vi "Perform Action.vi"(8 "error in":errorcluster, 10 "Input":variant, 11 "Red-y Read Write CFG in":refnum<class "Red-y Pressure Control CFG Simulated.lvclass">) -> (0 "error out":errorcluster, 2 "Output":variant, 3 "Red-y Read Write CFG out":refnum<class "Red-y Pressure Control CFG Simulated.lvclass">)   [LabVIEW 2023, in "Red-y Pressure Control CFG Simulated.lvclass"]
uses:
  Red-y Pressure Control CFG Simulated.lvclass
  Red-y Pressure Control CFG Simulated.lvclass/Red-y Pressure Control CFG Simulated.ctl
  <userlib>/_OpenG.lib/lvdata/lvdata.llb/Type Descriptor Enumeration__ogtk.ctl
  <userlib>/_OpenG.lib/lvdata/lvdata.llb/openg_variant.lvlib
  Pressure Control CFG/Read Write PE Input.ctl
  <vilib>/ErrorRing/Error Ring.xnode
  <vilib>/Utility/error.llb/Error Cluster From Error Code.vi
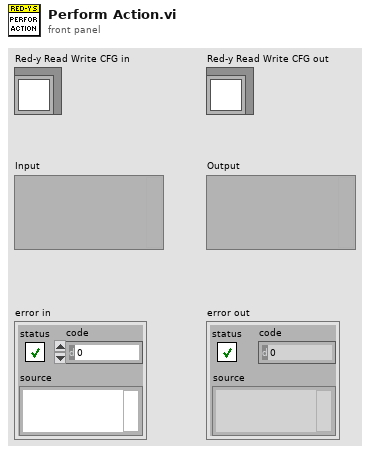
[diagram p1: front panel]
types:
  T1 = typedef "Read Write PE Input.ctl" = cluster{"Action":enum16{"Write", "Read"}, "Register":u16, "Type":T2, "Data":variant}
  T2 = typedef "openg_variant.lvlib/Type Descriptor Enumeration__ogtk.ctl" = enum8{"<Null>", "I8", "I16", "I32", "I64", "U8", "U16", "U32", "U64", "SGL", "DBL", "EXT", "CSG", "CDB", "CXT", "0x0F", "0x10", "0x11", "0x12", "0x13", "0x14", "Enum U8", "Enum U16", "Enum U32", "Enum U64", "SGL PQ", "DBL PQ", "EXT PQ", "CSG PQ", "CDB PQ", "CXT PQ", "0x1F", "0x20", "Boolean", "0x22", "0x23", "0x24", "0x25", "0x26", "0x27", "0x28", "0x29", "0x2A", "0x2B", "0x2C", "0x2D", "0x2E", "0x2F", "String", "0x31", "Path", "Pict", "0x34", "0x35", "0x36", "DAQ", "0x38", "0x39", "0x3A", "0x3B", "0x3C", "0x3D", "0x3E", "0x3F", "Array", "0x41", "0x42", "0x43", "0x44", "0x45", "0x46", "0x47", "0x48", "0x49", "0x4A", "0x4B", "0x4C", "0x4D", "0x4E", "0x4F", "Cluster", "0x51", "0x52", "Variant", "Waveform", "0x55", "0x56", "0x57", "0x58", "0x59", "0x5A", "0x5B", "0x5C", "0x5D", "0x5E", "Fixed Point", "0x60", "0x61", "0x62", "0x63", "0x64", "0x65", "0x66", "0x67", "0x68", "0x69", "0x6A", "0x6B", "0x6C", "0x6D", "0x6E", "0x6F", "Refnum", "0x71", "0x72", "Set Collection", "Map Collection"}
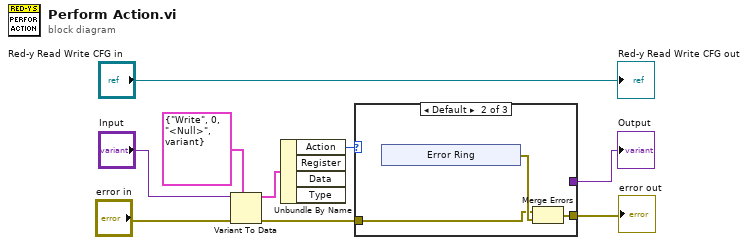
[diagram p0: block diagram]
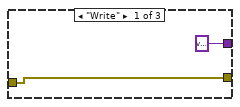
[diagram p2: hidden frame]
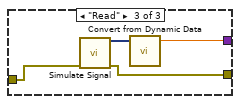
[diagram p3: hidden frame]
diagram:
  n1 = Variant To Data(error in="error in", type=T1 {"Action"=enum."Write", "Register"=0, "Type"=enum."<Null>", "Data"=variant}, Variant="Input") -> (data=w9:T1, error out=w4:errorcluster)
  n2 = Unbundle By Name(w9) -> ("Action"=w5:enum16{"Write", "Read"})  [unwired: 3 out]
  n3 = case shown="Default" w5 {
    tunnel: w4 -> [w11 w13 w23]
    tunnel: [w11 w12 w22] -> w3
    tunnel: [variant _ w20] -> w2
    frame "Write" {
    }
    frame Default {
      n4 = xnode "Error Ring"() -> ("error out"=w14:errorcluster)
      n5 = Merge Errors(w13, w14) -> (w12:errorcluster)
    }
    frame "Read" {
      n6 = call "Simulate Signal"("error in (no error)"=w23) -> ("Sine with Uniform Noise"=w21:dynamicdata, "error out"=w22:errorcluster)  [unwired: 13 in]
      n7 = call "Convert from Dynamic Data"("Dynamic Data Type"=w21) -> ("Scalar"=w20:dbl)  [unwired: 3 in]
    }
  }
  "error out" <- w3
  "Output" <- w2
  "Red-y Read Write CFG out" <- "Red-y Read Write CFG in"
